vi "Siren logic.vi"(7 "Data out":T1, 11 "Strobe Light State":bool) -> (3 "Siren State Out":bool)   [LabVIEW 2025, in "SafetyLight.lvlib"]
uses:
  SafetyLight.lvlib
  safety light settings.ctl
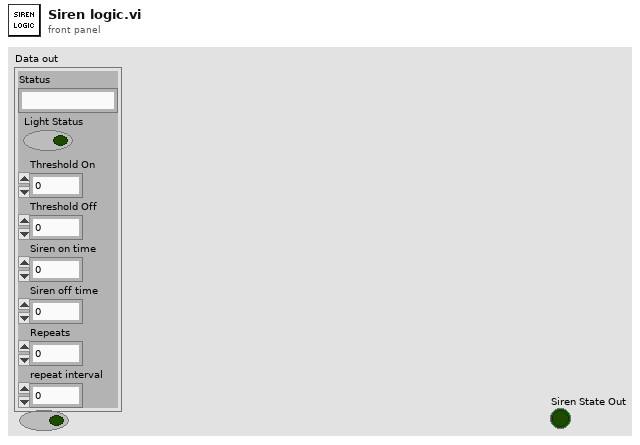
[diagram p1: front panel]
types:
  T1 = typedef "safety light settings.ctl" = cluster{"Status":string, "Light Status":bool, "Threshold On":dbl, "Threshold Off":dbl, "Siren on time":dbl, "Siren off time":dbl, "Repeats":i32, "repeat interval":dbl}
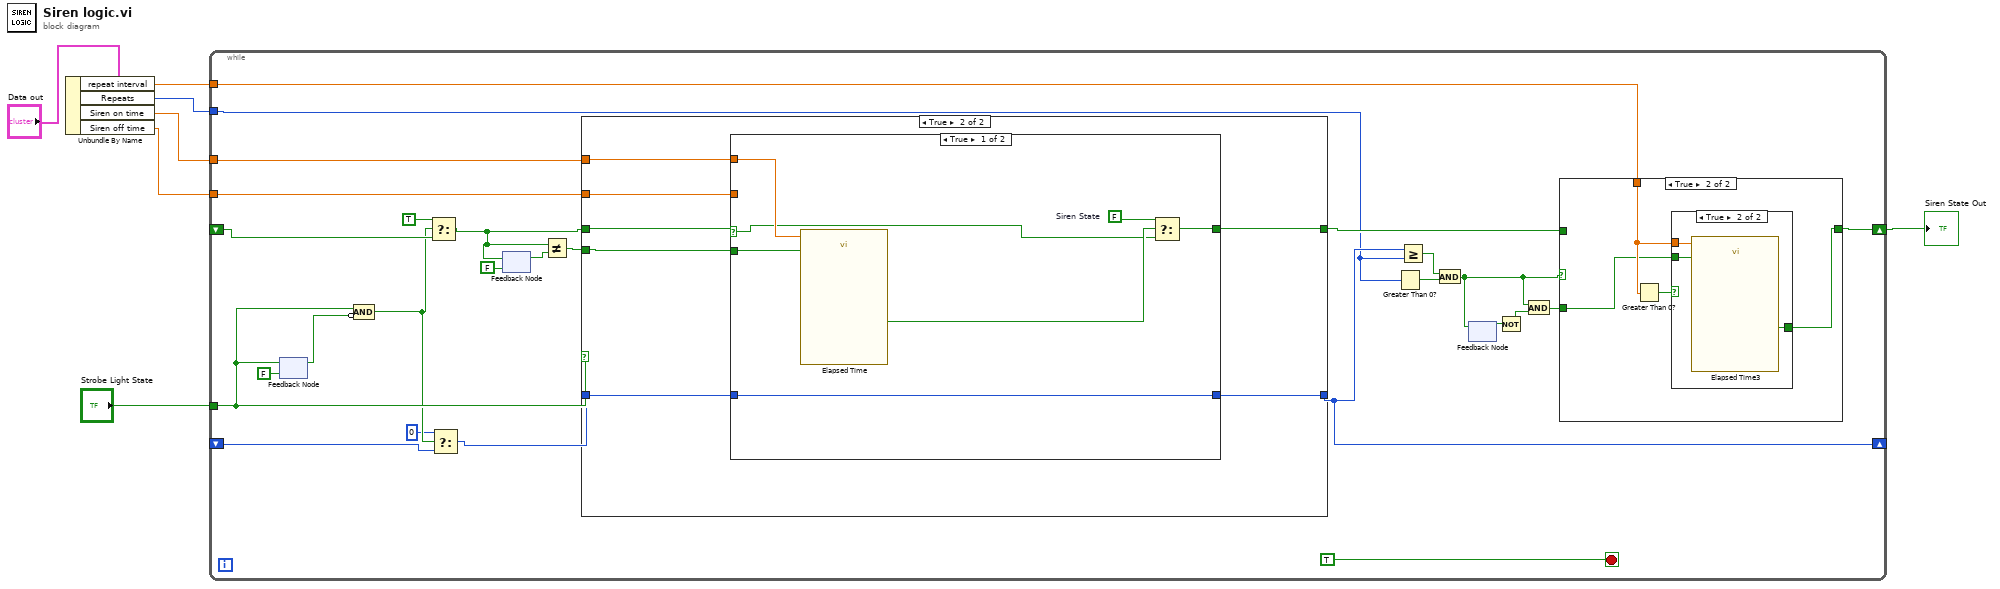
[diagram p0: block diagram]
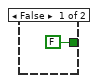
[diagram p3: hidden frame]
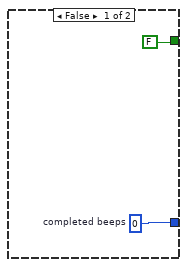
[diagram p4: hidden frame]
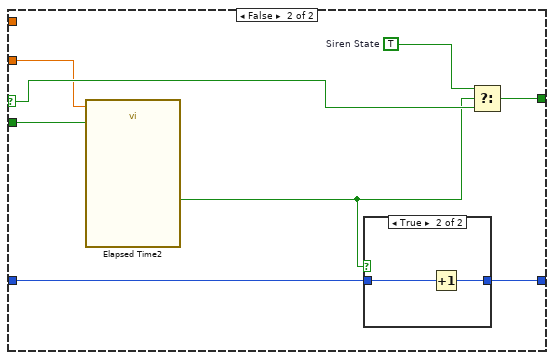
[diagram p5: hidden frame]
diagram:
  n1 = Unbundle By Name("Data out") -> ("repeat interval"=w1:dbl, "Repeats"=w4:i32, "Siren on time"=w3:dbl, "Siren off time"=w2:dbl)
  n2 = while {
    shift-right: [w31] -> _
    shift-left: _ -> [w17]
    tunnel: "Strobe Light State" -> [w23]
    tunnel: w4 -> [w13]
    tunnel: w3 -> [w33]
    tunnel: w2 -> [w32]
    shift-right: [w26] -> w6
    shift-left: _ -> [w22]
    tunnel: w1 -> [w12]
    stop <- TRUE stop-if-true
    n3 = feedback #1(FALSE ("Siren State")) -> (w24:bool)
    n4 = feedback-in #1(w23) -> ()
    n5 = Compound Arithmetic op=AND(w23, invert w24) -> (w19:bool)
    n6 = Select(t=TRUE, s=w19, f=w22) -> (s? t:f=w21:bool)
    n7 = Select(t=0, s=w19, f=w17) -> (s? t:f=w18:i32)
    n8 = feedback-in #2(w21) -> ()
    n9 = feedback #2(FALSE ("Siren State")) -> (w29:bool)
    n10 = Not Equal?(x=w21, y=w29) -> (x != y?=w28:bool)
    n11 = case shown="True" w23 {
      tunnel: [FALSE ("Siren State") w52] -> w27
      tunnel: w21 -> [_ w51]
      tunnel: w33 -> [_ w50]
      tunnel: [w44 w48] -> w31
      tunnel: w32 -> [_ w49]
      tunnel: w18 -> [_ w47]
      tunnel: w28 -> [_ w46]
      frame False {
        w44 = 0  # completed beeps
      }
      frame True {
        n12 = case shown="True" w51 {
          selector: w51 -> [w54 w64]
          tunnel: [w57 w66] -> w52
          tunnel: w46 -> [w59 w67]
          tunnel: w50 -> [w58 _]
          tunnel: w49 -> [_ w63]
          tunnel: [w53 w61] -> w48
          tunnel: w47 -> [w53 w60]
          frame True {
            w55 = FALSE  # Siren State
            n13 = call "Elapsed Time"("Time Target (s)"=w58, "Reset"=w59) -> ("Time has Elapsed"=w56:bool)  [unwired: 10 in, 7 out]
            n14 = Select(t=w55, s=w56, f=w54) -> (s? t:f=w57:bool)
          }
          frame False {
            w65 = TRUE  # Siren State
            n15 = call "Elapsed Time2"("Time Target (s)"=w63, "Reset"=w67) -> ("Time has Elapsed"=w62:bool)  [unwired: 10 in, 7 out]
            n16 = case shown="True" w62 {
              tunnel: w60 -> [w68 w70]
              tunnel: [w68 w69] -> w61
              frame False {
              }
              frame True {
                n17 = Increment(x=w70) -> (x+1=w69:i32)
              }
            }
            n18 = Select(t=w65, s=w62, f=w64) -> (s? t:f=w66:bool)
          }
        }
      }
    }
    n19 = Greater Than 0?(x=w13) -> (x > 0?=w14:bool)
    n20 = Greater Or Equal?(x=w31, y=w13) -> (x >= y?=w15:bool)
    n21 = And(x=w15, y=w14) -> (x .and. y?=w9:bool)
    n22 = feedback-in #3(w9) -> ()
    n23 = feedback #3() -> (w11:bool)  [unwired: 1 in]
    n24 = Not(x=w11) -> (.not. x?=w10:bool)
    n25 = And(x=w9, y=w10) -> (x .and. y?=w8:bool)
    n26 = case shown="True" w9 {
      tunnel: [w35 w37] -> w26
      tunnel: w27 -> [w35 _]
      tunnel: w12 -> [_ w38]
      tunnel: w8 -> [_ w36]
      frame False {
      }
      frame True {
        n27 = Greater Than 0?(x=w38) -> (x > 0?=w39:bool)
        n28 = case shown="True" w39 {
          tunnel: w38 -> [_ w43]
          tunnel: [FALSE ("Time has Elapsed") w42] -> w37
          tunnel: w36 -> [_ w41]
          frame False {
          }
          frame True {
            n29 = call "Elapsed Time3"("Time Target (s)"=w43, "Reset"=w41) -> ("Time has Elapsed"=w42:bool)  [unwired: 10 in, 7 out]
          }
        }
      }
    }
  }
  "Siren State Out" <- w6
